vi "read_halo_level.vi"   [LabVIEW 2016]
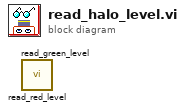
[diagram p0: block diagram]
diagram:
  n1 = call "read_red_level.vi"() -> ()  [unwired: 3 in, 2 out]
  n2 = call "read_green_level.vi"() -> ()  [unwired: 3 in, 2 out]
